vi "testStandardErrorBehavior.vi"() -> ()   [LabVIEW 2019, in "AssertionTest.lvlib"]
uses:
  AssertionTest.lvlib
  b47332d7-55f6-4b66-862f-220e59fed965.vi
  <vilib>/Utility/error.llb/Error Cluster From Error Code.vi
  Constraint/IsEqual/Create.vi
  <vilib>/ErrorRing/Error Ring.xnode
  Constraint/IsEqual/IsEqual.lvclass
panel:
  out "error out":errorcluster
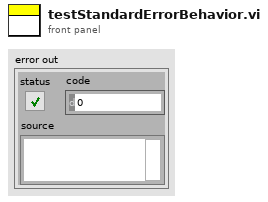
[diagram p1: front panel]
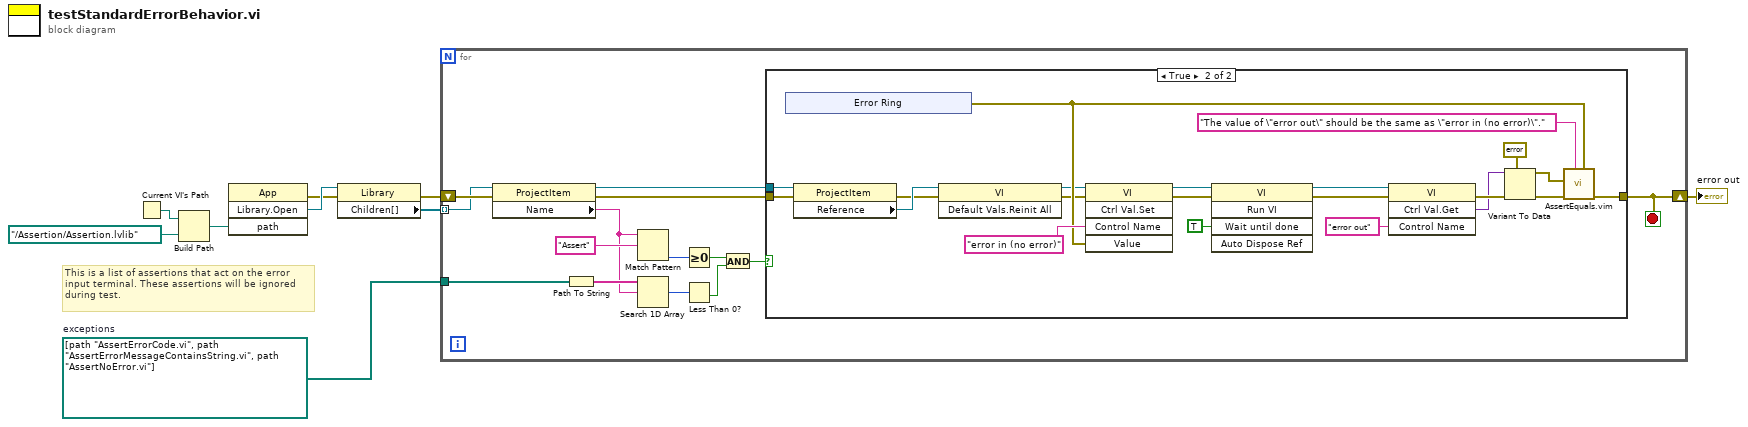
[diagram p0: block diagram]
diagram:
  w1 = path[] [path "AssertErrorCode.vi", path "AssertErrorMessageContainsString.vi", path "AssertNoError.vi"]  # exceptions
  # "This is a list of assertions that act on the error\ninput terminal. These assertions will be ignored\nduring test."
  n1 = Current VI's Path() -> (path=w8:path)
  n2 = Build Path(base path=w8, name or relative path=path "../Assertion/Assertion.lvlib") -> (appended path=w6:path)
  n3 = invoke class="App" method="Library.Open"("path"=w6) -> (error out=w4:errorcluster, "Open Library"=w5:refnum<vi>)  [unwired: 3 in, 2 out]
  n4 = property class="Library"(reference=w5, error in=w4) -> (error out=w2:errorcluster, "Children[]"=w3:refnum<vi>[])  [unwired: 1 out]
  n5 = for {
    tunnel: w3 -> [w22] mode=indexing
    tunnel: w1 -> [w17]
    shift-right: [w18] -> w9
    shift-left: w2 -> [w23]
    stop <- w18 stop-if-true
    n6 = property class="ProjectItem"(reference=w22, error in=w23) -> (reference out=w20:refnum<vi>, error out=w19:errorcluster, "Name"=w15:string)
    n7 = Path To String(path=w17) -> (string=w16:string[])
    n8 = Match Pattern(string=w15, regular expression="Assert") -> (offset past match=w14:i32)  [unwired: 1 in, 3 out]
    n9 = Search 1D Array(1D array=w16, element=w15) -> (index of element=w12:i32)  [unwired: 1 in]
    n10 = Greater Or Equal To 0?(x=w14) -> (x >= 0?=w13:bool)
    n11 = Less Than 0?(x=w12) -> (x < 0?=w11:bool)
    n12 = And(x=w13, y=w11) -> (x .and. y?=w10:bool)
    n13 = case shown="True" w10 {
      tunnel: w20 -> [_ w31]
      tunnel: w19 -> [w24 w30]
      tunnel: [w24 w37] -> w18
      frame False {
      }
      frame True {
        n14 = xnode "Error Ring"() -> ("error out"=w36:errorcluster)
        n15 = property class="ProjectItem"(reference=w31, error in=w30) -> (error out=w25:errorcluster, "Reference"=w26:refnum<vi>)  [unwired: 1 out]
        n16 = invoke class="VI" method="Default Vals.Reinit All"(reference=w26, error in=w25) -> (reference out=w27:refnum<vi>, error out=w28:errorcluster)  [unwired: 1 in, 1 out]
        n17 = invoke class="VI" method="Ctrl Val.Set"(reference=w27, error in=w28, "Control Name"="error in (no error)", "Value"=w36) -> (reference out=w43:refnum<vi>, error out=w44:errorcluster)  [unwired: 1 in, 3 out]
        n18 = invoke class="VI" method="Run VI"(reference=w43, error in=w44, "Wait until done"=TRUE ("Wait Until Done")) -> (reference out=w40:refnum<vi>, error out=w41:errorcluster)  [unwired: 2 in, 3 out]
        n19 = invoke class="VI" method="Ctrl Val.Get"(reference=w40, error in=w41, "Control Name"="error out") -> (error out=w38:errorcluster, "Get Control Value Variant"=w34:variant)  [unwired: 1 in, 2 out]
        n20 = Variant To Data(error in=w38, type=errorcluster {"status"=FALSE, "code"=0, "source"=""} ("error constant"), Variant=w34) -> (data=w32:errorcluster, error out=w35:errorcluster)
        n21 = call "AssertEquals.vim"("Expected"=w36, "Message (\"\")"="The value of \"error out\" should be the same as \"error in (no error)\"." ("Message (\"\")"), "error in (no error)"=w35, "Actual"=w32) -> ("error out"=w37:errorcluster)  [unwired: 7 in]
      }
    }
  }
  "error out" <- w9
